vi "SwissSPAD Live_Get Control Label & Settings Element.vi"(8 "Error In":errorcluster, 11 "CtlRef":refnum<vi>) -> (0 "Error Out":errorcluster, 1 "Control Label":string, 3 "Settings Element":T1)   [LabVIEW 2021]
uses:
  SwissSPAD Live_Settings List.ctl
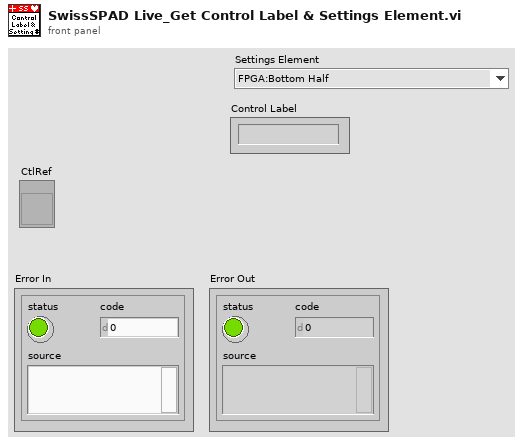
[diagram p1: front panel]
types:
  T1 = typedef "SwissSPAD Live_Settings List.ctl" = enum16{"FPGA:Bottom Half", "FPGA:Top Half", "FPGA:Bottom Bitfile Path", "FPGA:Top Bitfile Path", "FPGA:Bottom Bitstream Version", "FPGA:Top Bitstream Version", "FPGA:Auto Reset FPGA", "FPGA:Bottom FPGA Serial Number", "FPGA:Top FPGA Serial Number", "FPGA:Detector PCB Version", "Acquisition Parameters:Microlens", "Acquisition Parameters:SS2 DAQ Parameters", "Acquisition Parameters:Gate Configuration Array", "Acquisition Parameters:SS3 DAQ Parameters", "Acquisition Parameters:Buffer Size (# 8-bit Gates)", "File Information:File Information", "File Information:# Datasets in Series", "File Information:Scrambled File Flag", "File Information:SS3 Gate Slip Correction", "File Information:SS3 Hot Pixel Mismatch Detection", "File Information:Delay between Datasets", "File Information:Save Sum of All Gates Preview", "Image Parameters:Image ROI Information", "Image Parameters:Image Binning Options", "Image Parameters:SS3 Displayed Image", "Image Parameters:Image Display Options", "Image Parameters:Use Histogram Cursors", "Image Parameter:FPGA Data to Display", "UI Settings:Histogram Bins Number", "UI Settings:Histogram Bin Size", "UI Settings:Use Image Display Options", "UI Settings:Verbose Settings", "UI Settings:Verbose Saving"}
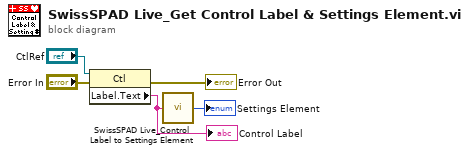
[diagram p0: block diagram]
diagram:
  n1 = property class="Ctl"(reference="CtlRef", error in="Error In") -> (error out=→"Error Out":errorcluster, "Label.Text"=w2:string)  [unwired: 1 out]
  "Control Label" <- w2
  n2 = call "SwissSPAD Live_Control Label to Settings Element.vi"("Control Label"=w2) -> ("Settings List Element"=→"Settings Element":T1)  [unwired: 8 in]
